vi "TalonSRXReadEncoder.vi"(0 "Device Reference (in)":T1, 1 "Gear Ratio":dbl=1.0, 5 "Simulated Position Goal (deg)":dbl, 7 "Simulated Velocity (deg/s)":dbl=50.0 format="%#_13g", 9 "Simulate":bool, 11 "Error (in)":errorcluster) -> (4 "Device Reference (out)":T1, 6 "Position (deg)":dbl, 8 "Velocity (deg/s)":dbl, 15 "Error (out)":errorcluster)   [LabVIEW 2020]
doc: "Wrapper for reading the integrated encoders from a Talon SRX motor controller. Provides support for simulating the postion of the motor."
uses:
  <vilib>/Rock Robotics/WPI/MotorControl/WPI_MotorControlDeviceRef.ctl
  <vilib>/Rock Robotics/WPI/MotorControl/WPI_MotorControlType.ctl
  <vilib>/Rock Robotics/SystemInterfaces/DIO/FPGA_DIOPWMChannel.ctl
  <vilib>/Rock Robotics/WPI/PWM/WPI_PWMDeadband.ctl
  <vilib>/Rock Robotics/SystemInterfaces/DIO/FPGA_DIOChannel.ctl
  <vilib>/Rock Robotics/WPI/ThirdParty/Phoenix-LabVIEW/Motor Controller/Get/CTRE_Phoenix_MotorController_GetSelectedSensorData.vi
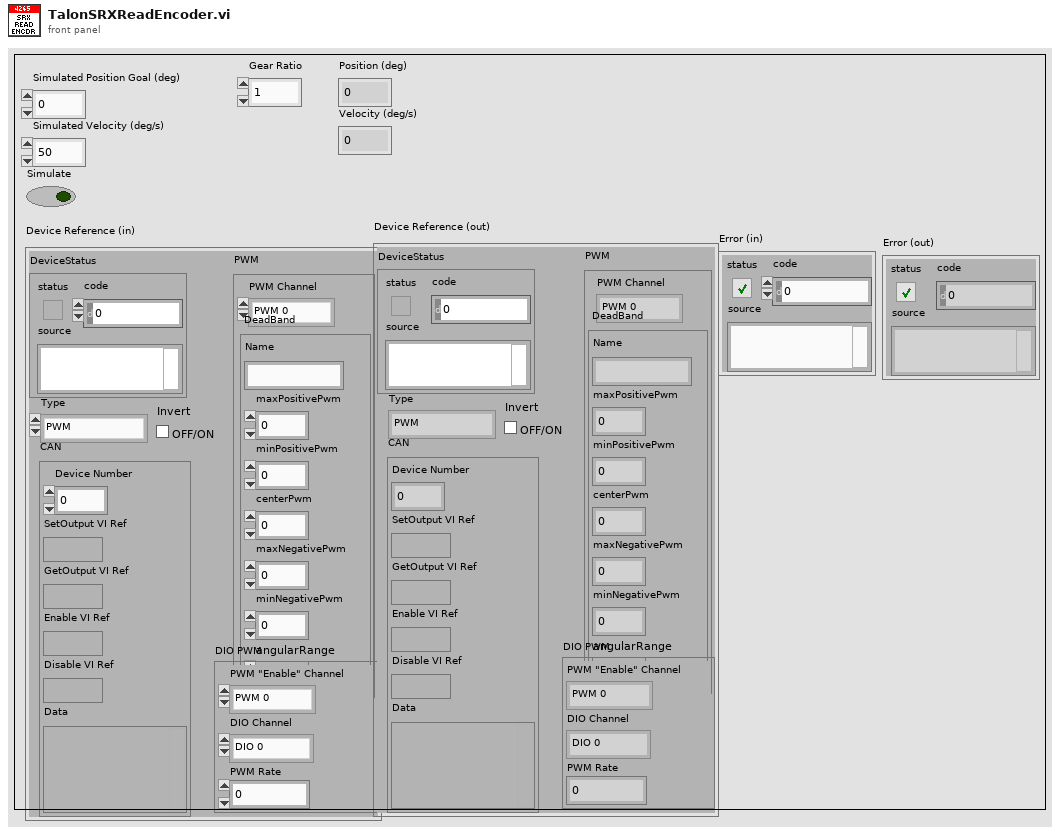
[diagram p1: front panel]
types:
  T1 = typedef "WPI_MotorControlDeviceRef.ctl" = cluster{"DeviceStatus":errorcluster, "Type":T2, "PWM":cluster{"PWM Channel":T3, "DeadBand":T4}, "CAN":cluster{"Device Number":u8, "SetOutput VI Ref":variant, "GetOutput VI Ref":variant, "Enable VI Ref":variant, "Disable VI Ref":variant, "Data":variant}, "Invert":bool, "DIO PWM":cluster{"PWM \"Enable\" Channel":T3, "DIOChannel":T5, "PWM Rate":dbl}}
  T2 = typedef "WPI_MotorControlType.ctl" = enum16{"PWM", "CAN", "DIO PWM"}
  T3 = typedef "FPGA_DIOPWMChannel.ctl" = enum8{"PWM 0", "PWM 1", "PWM 2", "PWM 3", "PWM 4", "PWM 5", "PWM 6", "PWM 7", "PWM 8", "PWM 9", "PWM MXP 0", "PWM MXP 1", "PWM MXP 2", "PWM MXP 3", "PWM MXP 4", "PWM MXP 5", "PWM MXP 6", "PWM MXP 7", "PWM MXP 8", "PWM MXP 9", "Invalid"}
  T4 = typedef "WPI_PWMDeadband.ctl" = cluster{"Name":string, "maxPositivePwm":i32, "minPositivePwm":i32, "centerPwm":i32, "maxNegativePwm":i32, "minNegativePwm":i32, "angularRange":u16}
  T5 = typedef "FPGA_DIOChannel.ctl" = enum8{"DIO 0", "DIO 1", "DIO 2", "DIO 3", "DIO 4", "DIO 5", "DIO 6", "DIO 7", "DIO 8", "DIO 9", "DIO MXP 0", "DIO MXP 1", "DIO MXP 2", "DIO MXP 3", "DIO MXP 4", "DIO MXP 5", "DIO MXP 6", "DIO MXP 7", "DIO MXP 8", "DIO MXP 9", "DIO MXP 10", "DIO MXP 11", "DIO MXP 12", "DIO MXP 13", "DIO MXP 14", "DIO MXP 15", "SPI Port CS1", "SPI Port CS2", "SPI Port CS3", "SPI Port MISO", "SPI Port MOSI", "Invalid"}
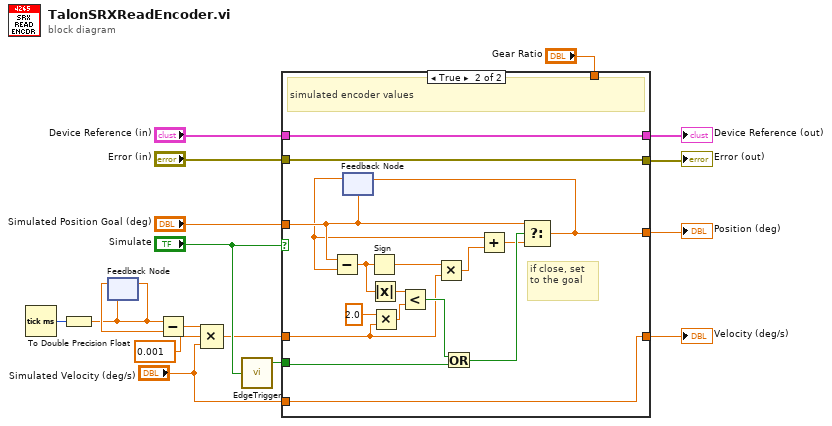
[diagram p0: block diagram]
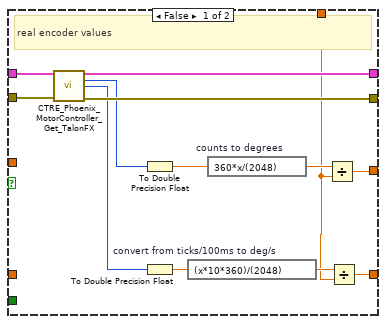
[diagram p2: hidden frame]
diagram:
  n1 = Tick Count (ms)() -> (millisecond timer value=w7:u32)
  n2 = To Double Precision Float(number=w7) -> (double precision float=w5:dbl)
  n3 = feedback-in #1(w5) -> ()
  n4 = feedback #1(w5) -> (w6:dbl)
  n5 = Subtract(x=w5, y=w6) -> (x-y=w4:dbl)
  n6 = Compound Arithmetic op=MULTIPLY(w4, 0.001 ("value"), "Simulated Velocity (deg/s)") -> (w2:dbl)
  n7 = call "EdgeTrigger.vi"("Input Signal"="Simulate") -> ("Rising Edge Trigger"=w14:bool)  [unwired: 2 out]
  n8 = case shown="True" "Simulate" {
    tunnel: [w30 w35] -> w11
    tunnel: [w29 w34] -> w12
    tunnel: [w23 w33] -> w9
    tunnel: [w19 w31] -> w8
    tunnel: "Device Reference (in)" -> [w28 w35]
    tunnel: "Error (in)" -> [w27 w34]
    tunnel: w14 -> [_ w47]
    tunnel: "Simulated Position Goal (deg)" -> [_ w46]
    tunnel: "Gear Ratio" -> [w18 _]
    tunnel: w2 -> [_ w32]
    tunnel: "Simulated Velocity (deg/s)" -> [_ w31]
    frame False {
      # "real encoder values"
      n9 = call-poly <vilib>:"CTRE_Phoenix_MotorController_Get_TalonFX.vi"("PhoenixMotorControlDevRef"=w28, "error in"=w27) -> ("PhoenixMotorControlDevRef"=w30:T1, "Position (Raw Sensor Units)"=w24:i32, "Velocity (Raw Sensor Units per 100 ms)"=w20:i32, "error out"=w29:errorcluster)  [unwired: 10 in]
      n10 = To Double Precision Float(number=w24) -> (double precision float=w25:dbl)
      n11 = To Double Precision Float(number=w20) -> (double precision float=w22:dbl)
      n12 = expression code="(x*10*360)/(2048)" "convert from ticks/100ms to deg/s"(w22) -> (w21:dbl)
      n13 = expression code="360*x/(2048)" "counts to degrees"(w25) -> (w26:dbl)
      n14 = Divide(x=w26, y=w18) -> (x/y=w23:dbl)
      n15 = Divide(x=w21, y=w18) -> (x/y=w19:dbl)
    }
    frame True {
      # "if close, set\nto the goal"
      # "simulated encoder values"
      n16 = feedback #2(w46) -> (w41:dbl)
      n17 = Subtract(x=w46, y=w41) -> (x-y=w40:dbl)
      n18 = Sign(1:w40) -> (0:w43:dbl)
      n19 = Absolute Value(x=w40) -> (abs(x)=w39:dbl)
      n20 = Multiply(x=2.0, y=w32) -> (x*y=w38:dbl)
      n21 = Less?(x=w39, y=w38) -> (x < y?=w45:bool)
      n22 = Multiply(x=w43, y=w32) -> (x*y=w42:dbl)
      n23 = Or(x=w45, y=w47) -> (x .or. y?=w44:bool)
      n24 = Add(x=w41, y=w42) -> (x+y=w36:dbl)
      n25 = Select(t=w46, s=w44, f=w36) -> (s? t:f=w33:dbl)
      n26 = feedback-in #2(w33) -> ()
    }
  }
  "Position (deg)" <- w9
  "Velocity (deg/s)" <- w8
  "Error (out)" <- w12
  "Device Reference (out)" <- w11
